vi "Replace Object Constant Labels.vi"(6 "Post":string, 8 "error in":errorcluster, 9 "Pre":string, 10 "VI Ref":refnum<vi>) -> (0 "error out":errorcluster)   [LabVIEW 2021, in "_Rename.lvlib" / "_Rename.lvclass"]
uses:
  _Rename.lvclass
  _Rename.lvclass/_Rename.ctl
  <vilib>/Utility/traverseref.llb/TRef TravTarget.ctl
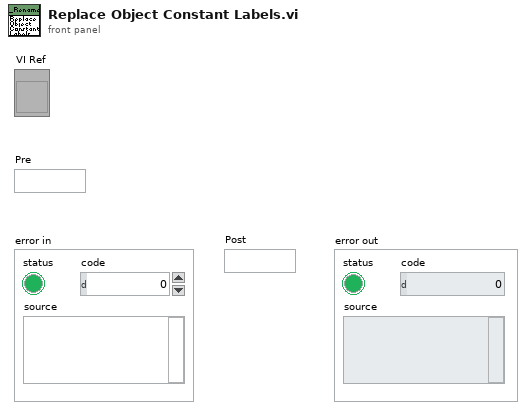
[diagram p1: front panel]
types:
  T1 = typedef "TRef TravTarget.ctl" = enum16{"FP", "BD", "Other"}
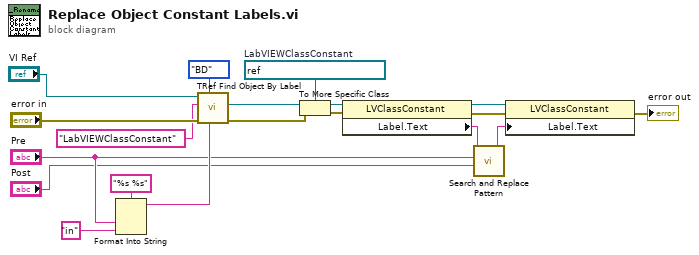
[diagram p0: block diagram]
diagram:
  w7 = refnum<vi> refnum  # LabVIEWClassConstant
  n1 = Format Into String(format string="%s %s", "Pre", "in" ("input 2")) -> (resulting string=w17:string)  [unwired: 2 in, 1 out]
  n2 = call <vilib>:"TRef Find Object By Label.vi"("Label"=w17, "Traverse Target"=TRef_TravTarget."BD", "error in (no error)"="error in", "Class Name"="LabVIEWClassConstant", "VI Ref"="VI Ref") -> ("error out"=w16:errorcluster, "Found Obj Ref"=w19:refnum<vi>)  [unwired: 3 in, 2 out]
  n3 = To More Specific Class(target class=w7, reference=w19, error in=w16) -> (specific class reference=w6:refnum<vi>, error out=w5:errorcluster)
  n4 = property class="LVClassConstant"(reference=w6, error in=w5) -> (reference out=w3:refnum<vi>, error out=w4:errorcluster, "Label.Text"=w2:string)
  n5 = call <vilib>:"Search and Replace Pattern.vi"("string"=w2, "regular expression (\"\")"="Pre", "replace string (\"\")"="Post") -> ("result string"=w1:string)  [unwired: 2 in, 1 out]
  n6 = property class="LVClassConstant"(reference=w3, error in=w4, "Label.Text"=w1) -> (error out=→"error out":errorcluster)  [unwired: 1 out]
